vi "test4-ArgumentCanBeTakenToTargetModule.vi"(8 "error in (no error)":errorcluster, 11 "TestCase in":refnum<class "testcase-CSMArgument.lvclass">) -> (0 "error out":errorcluster, 3 "TestCase out":refnum<class "testcase-CSMArgument.lvclass">)   [LabVIEW 2017, in "testcase-CSMArgument.lvclass"]
uses:
  testcase-CSMArgument.lvclass
  a780a543-d55d-4312-9572-3fc81e4783fb.vi
  <vilib>/addons/_JKI Toolkits/VI Tester/TestCase.llb/TestCase.lvclass
  src/user.lib/_NEVSTOP/Communicable State Machine(CSM)/Communicable State Machine.lvlib
  CSM/CSM-Testcase.lvlib
  C:/Program Files (x86)/National Instruments/LabVIEW 2017/vi.lib/addons/_JKI Toolkits/VI Tester/TestCase.llb/TestCase.lvclass
panel:
  out "LoopCount":i32
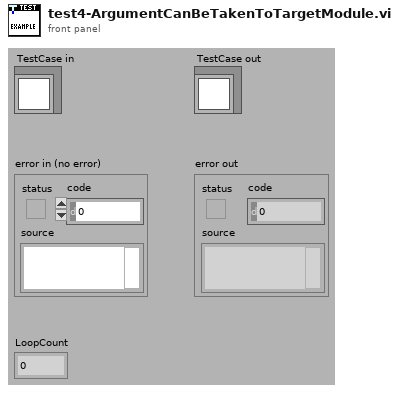
[diagram p1: front panel]
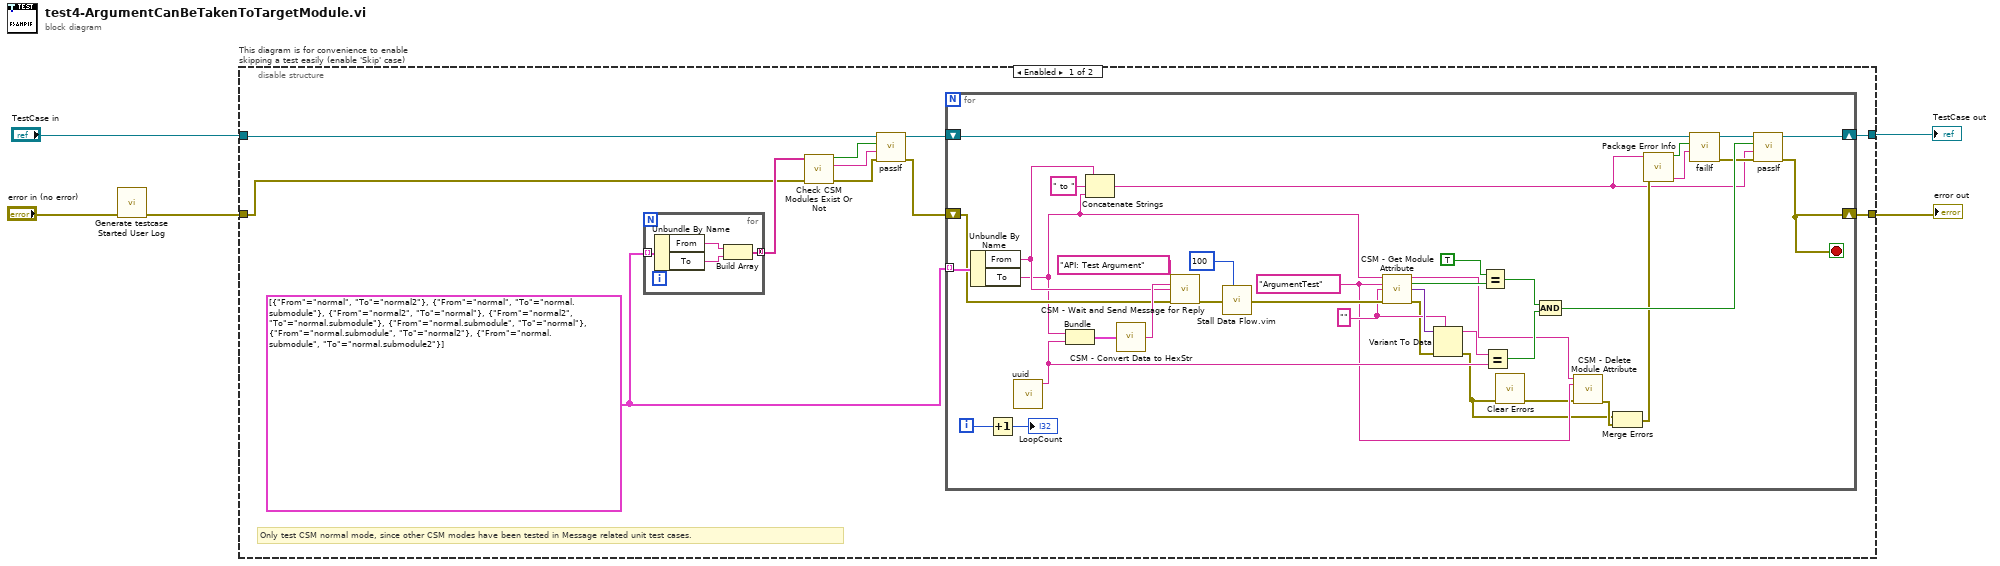
[diagram p0: block diagram]
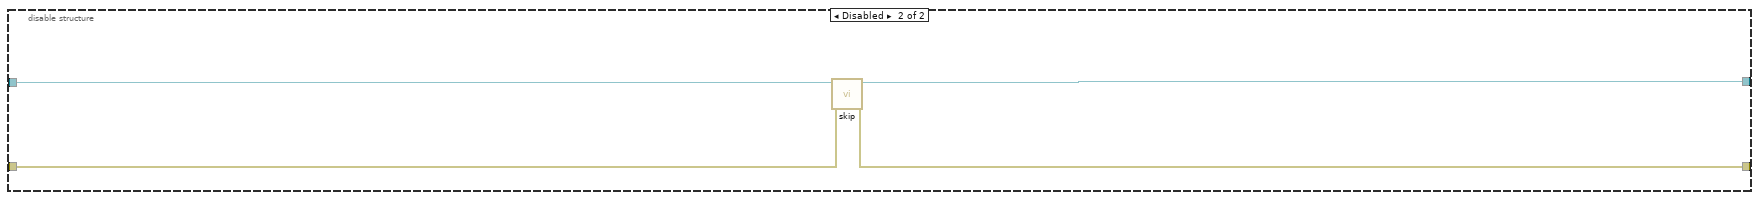
[diagram p2: hidden frame]
diagram:
  n1 = call "Generate testcase Started User Log.vi"("Error In"="error in (no error)") -> ("error out"=w1:errorcluster)  [unwired: 10 in]
  n2 = disable-structure "This diagram is for convenience to enable skipping a test easily (enable 'Skip' case)" shown="Enabled" {
    disable-tunnel: "TestCase in" -> [w9 w61]
    disable-tunnel: [w16 w59] -> w2
    disable-tunnel: [w15 w60] -> w4
    disable-tunnel: w1 -> [w7 w58]
    frame Enabled {
      w10 = cluster{"From":string, "To":string}[] [{"From"="normal", "To"="normal2"}, {"From"="normal", "To"="normal.submodule"}, {"From"="normal2", "To"="normal"}, {"From"="normal2", "To"="normal.submodule"}, {"From"="normal.submodule", "To"="normal"}, {"From"="normal.submodule", "To"="normal2"}, {"From"="normal.submodule", "To"="normal.submodule2"}]
      # "Only test CSM normal mode, since other CSM modes have been tested in Message related unit test cases."
      n3 = for {
        tunnel: w10 -> [w20] mode=indexing
        tunnel: [w17] -> w13 mode=concatenating
        n4 = Unbundle By Name(w20) -> ("From"=w19:string, "To"=w18:string)
        n5 = Build Array(w19, w18) -> (w17:string[])
      }
      n6 = call "Check CSM Modules Exist Or Not.vi"("error in"=w7, "CSM names in"=w13) -> ("error out"=w11:errorcluster, "Debug string"=w12:string, "All Modules Exist?"=w14:bool)  [unwired: 7 in]
      n7 = call-dynamic "passIf.vi"("error in (no error)"=w11, "message (\"\")"=w12, "pass"=w14, "TestCase in"=w9) -> ("error out"=w6:errorcluster, "TestCase out"=w8:refnum<class "testcase-CSMArgument.lvclass">)  [unwired: 6 in]
      n8 = for {
        tunnel: w10 -> [w57] mode=indexing
        shift-right: [w43] -> w16
        shift-left: w8 -> [w27]
        shift-right: [w42] -> w15
        shift-left: w6 -> [w34]
        i -> [w41]
        stop <- w42 stop-if-true
        w47 = ""
        w35 = "ArgumentTest" ("Attribute")
        n9 = Unbundle By Name(w57) -> ("From"=w32:string, "To"=w30:string)
        n10 = Increment(x=w41) -> (x+1=→"LoopCount":i32)
        n11 = call "uuid.vi"() -> ("UUID"=w45:string)  [unwired: 11 in]
        n12 = Bundle("To"=w30, "UUID"=w45) -> (w52:cluster{"To":string, "UUID":string})  [unwired: 1 in]
        n13 = Concatenate Strings(w32, " to " ("string"), w30) -> (w21:string)
        n14 = call "CSM - Convert Data to HexStr.vi"("Variant"=w52) -> ("HEX String (0-9,A-F)"=w51:string)  [unwired: 8 in]
        n15 = call "CSM - Wait and Send Message for Reply.vi"("State"="API: Test Argument", "Arguments (\"\")"=w51, "Target Module"=w32, "Error In (No Error)"=w34) -> ("error out"=w55:errorcluster)  [unwired: 8 in, 3 out]
        n16 = call "Stall Data Flow.vim"("value in"=w55, "milliseconds to wait"=u32 100) -> ("value out"=w53:errorcluster)  [unwired: 1 out]
        n17 = call "CSM - Get Module Attribute.vi"("CSM Name"=w30, "Attribute"=w35, "Default Value (Empty Variant)"=w47, "Error In"=w53) -> ("CSM Name (Dup)"=w36:string, "Found"=w50:bool, "Value"=w48:variant, "error out"=w44:errorcluster)  [unwired: 7 in, 1 out]
        n18 = Variant To Data(error in=w44, type=w47, Variant=w48) -> (data=w46:string, error out=w23:errorcluster)
        n19 = Equal?(x=TRUE, y=w50) -> (x = y?=w39:bool)
        n20 = Equal?(x=w46, y=w45) -> (x = y?=w38:bool)
        n21 = call <vilib>:"Clear Errors.vi"("error in (no error)"=w23) -> ("error out"=w33:errorcluster)  [unwired: 5 in, 1 out]
        n22 = Compound Arithmetic op=AND(w39, w38) -> (w37:bool)
        n23 = call "CSM - Delete Module Attribute.vi"("CSM Name"=w36, "Attribute"=w35, "Error In"=w33) -> ("error out"=w24:errorcluster)  [unwired: 9 in, 3 out]
        n24 = Merge Errors(w23, w24) -> (w22:errorcluster)
        n25 = call "Package Error Info.vi"("error in"=w22, "String in"=w21) -> ("packed error info out"=w28:string, "error status"=w29:bool)  [unwired: 8 in]
        n26 = call-dynamic "failIf.vi"("message (\"\")"=w28, "fail"=w29, "TestCase in"=w27) -> ("error out"=w25:errorcluster, "TestCase out"=w26:refnum<class "testcase-CSMArgument.lvclass">)  [unwired: 7 in]
        n27 = call-dynamic "passIf.vi"("error in (no error)"=w25, "message (\"\")"=w21, "pass"=w37, "TestCase in"=w26) -> ("error out"=w42:errorcluster, "TestCase out"=w43:refnum<class "testcase-CSMArgument.lvclass">)  [unwired: 6 in]
      }
    }
    frame Disabled {
      # "skip test result while test is under development"
      n28 = call <vilib>:"skip.vi"("error in (no error)"=w58, "TestCase in"=w61) -> ("error out"=w60:errorcluster, "TestCase out"=w59:refnum<class "testcase-CSMArgument.lvclass">)  [unwired: 8 in]
    }
  }
  "error out" <- w4
  "TestCase out" <- w2
